vi "global_cms.vi"() -> ()   [LabVIEW 2015]
panel:
  in  "timeReset":u32
  in  "button":T1
  in  "mvs":T2
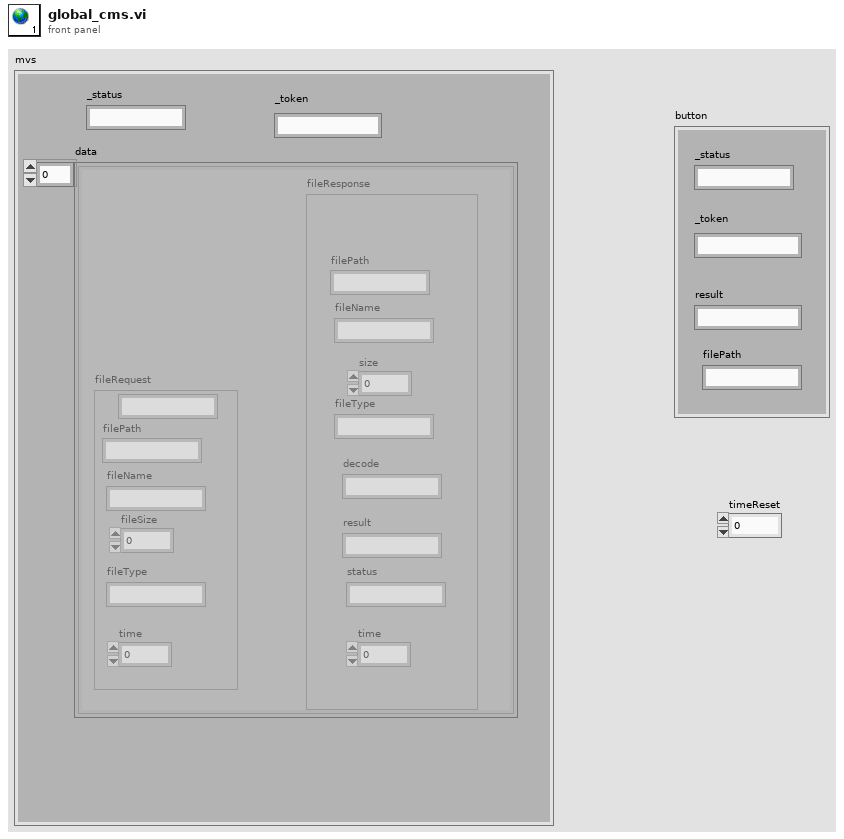
[diagram p1: front panel]
types:
  T1 = cluster{"_status":string, "_token":string, "result":string, "filePath":string}
  T2 = cluster{"data":cluster{"fileRequest":cluster{"filePath":string, "fileType":string, "fileName":string, "time":u32, "filePathTmp":string, "fileSize":u32}, "fileResponse":cluster{"filePath":string, "fileType":string, "fileName":string, "decode":string, "result":string, "status":string, "time":u32, "size":u32}}[], "_status":string, "_token":string}
diagram:
